vi "niUSRP EX QAM Tx student.vi"() -> ()   [LabVIEW 2020]
doc: "This example <B>requires the Modulation Toolkit</B>.\n\nApplies QAM (Quadrature Amplitude Modulation) to a PN sequence for USRP-based transmission. Continuously transmits a repeating message with a length determined by the PN Sequence Order parameter. \n\nThis example is paired with the example \"niUSRP Ex QAM Rx.vi\", which allows you to establish a Tx / Rx link between two separate USRPs. \n\nTo establish a Tx / Rx link between two USRPs:\n1) Ensure that the Tx and Rx example VIs have matching parameters for Modulation Scheme (M-Ary), Carrier Frequency, and Symbol Rate. Specify the Symbol Rate by setting the combination of the IQ Sampling Rate and the Number of Samples per Symbol parameters.\n2) Choose an IQ Sample Rate that enables sufficient Rx bandwidth.\n3) Set the Tx and / or Rx gain to ensure a sufficient signal to noise ratio on the Receive side. Note: applying too much gain can result in clipping.\n4) Choose a sufficient acquisition frame length that enables the demodulator to lock to the transmitted signal. National Instruments recommends that the acquired frame contain a number of symbols that is at least 20 * M-Ary of the modulation scheme. \n5) Ensure that the Reset Demodulator control is set to True until a solid lock is established. \n6) Install antennas and attenuators that efficiently operate at the carrier frequency you choose."
uses:
  <instrlib>/niUSRP/niUSRP Write Tx Data (CDB Cluster).vi
  <vilib>/addons/Modulation/niDMT.lvlib
panel:
  out "error out":errorcluster
  in  "Enabled Channel":string(combo)="0"
  out "Gain [dB] (actual)":dbl format="%#.6p"
  out "Carrier Frequency \n[Hz] (actual)":dbl=915000000.0 format="%#.6p"
  out "IQ Sampling\nRate [S/sec] (actual)":dbl=500000.0 format="%#.6p"
  in  "Active Antenna":string(combo)="TX1"
  in  "Gain [dB]":dbl format="%#.6p"
  in  "Carrier\nFrequency [Hz]":dbl=915000000.0 format="%#.6p"
  in  "IQ Sampling\nRate [S/sec]":dbl=500000.0 format="%#.6p"
  in  "Device Name":refnum<k15>="192.168.10.5"
  out "Frame Length [samples]":i32=2044
  in  "Pn Sequence Order":i32=13
  in  "Filter Parameters":T1={"Alpha"=0.5, "Filter Length"=6, "TX Filter"=enum."Root Raised Cos"} caption="Pulse Shaping Filter" {"Alpha" format="%.2f"}
  in  "QAM M-Ary":enum16{"4", "8", "16", "32", "64", "128", "256"}(ring)=enum."16"
  out "Symbol Rate [symbols/sec]":dbl=500000.0 format="%#.6p"
  in  "Samples Per Symbol":i32=4 min=2 step=2
  in  "Stop":bool
  out "Constellation Graph":T2(graph) caption="Tx Signal Constellation"
  # "Note:\nFrame size (samples per write) =\n (2^Pn Sequence Order) * Samples Per Symbol.\nUse Pn Sequence Order of 12 when using a 1 Gb Ethernet connection on a USRP RIO device. This prevents underflows by implicitly choosing \na frame size close to the ideal frame size for Ethernet connection. Refer to the \"Data Streaming Performance Tips\" section in the NI-USRP Help at ni.com/manuals for more information."
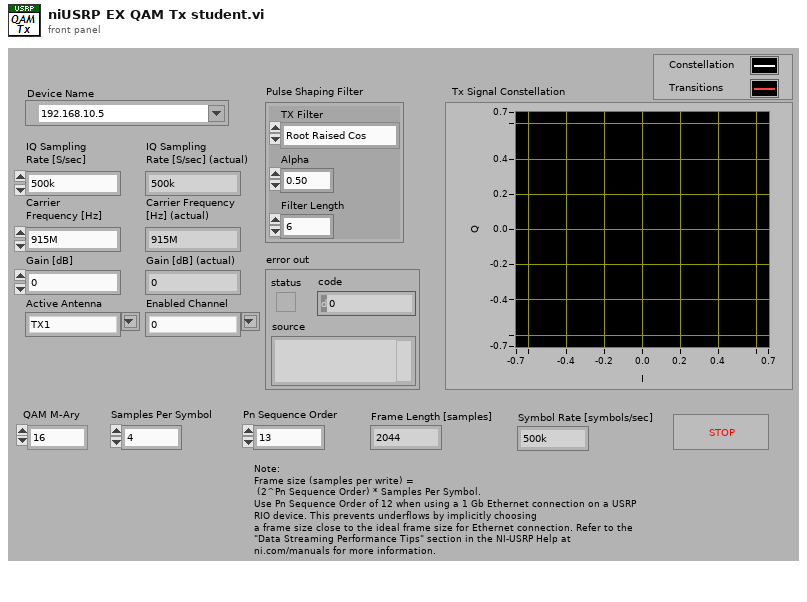
[diagram p1: front panel]
types:
  T1 = cluster{"Alpha":dbl, "Filter Length":i32, "TX Filter":enum16{"none", "Raised Cosine", "Root Raised Cos", "Gaussian"}}
  T2 = cluster{"constellation":dbl[], "oversampled data":dbl[]}[]
  T3 = enum32{"PN sequence", "User-defined pattern", "Read from file"}
  T4 = typedef "niAMT.lvlib/Complex Data Waveform.ctl" = cluster{"t0":dbl, "dt":dbl, "Y":cdb[]}
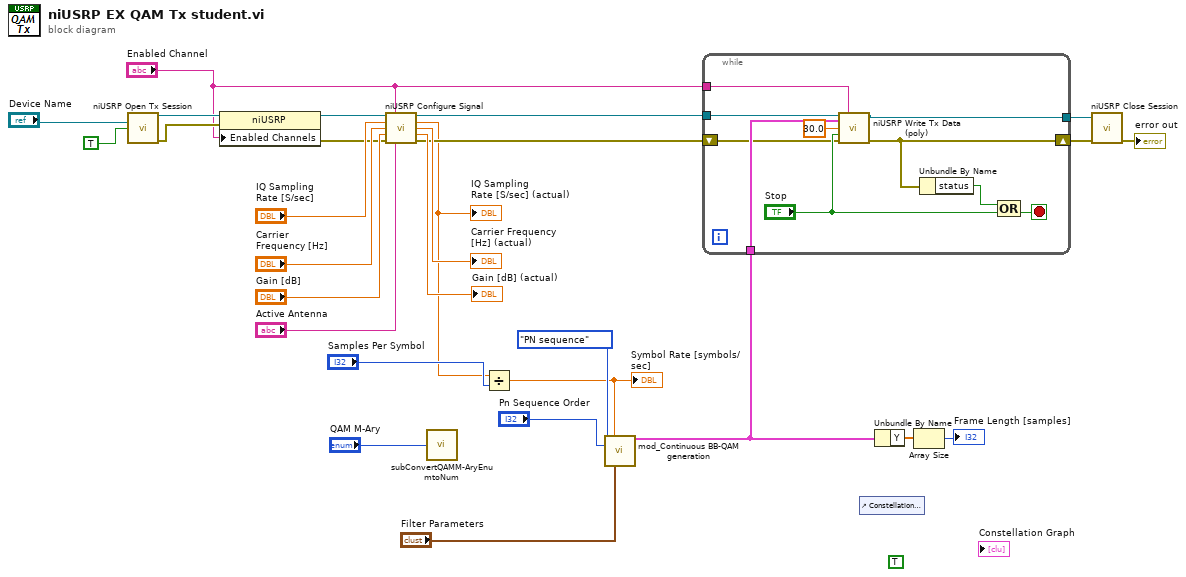
[diagram p0: block diagram]
diagram:
  (unwired) TRUE ("autoscale")
  n1 = call <instrlib>:"niUSRP Open Tx Session.vi"("device names"="Device Name", "reset"=TRUE) -> ("session handle out"=w6:refnum<k15>, "error out"=w4:errorcluster)  [unwired: 12 in]
  n2 = property class="niUSRP"(reference=w6, error in=w4, "Enabled Channels"="Enabled Channel") -> (reference out=w5:refnum<k15>, error out=w3:errorcluster)
  n3 = call <instrlib>:"niUSRP Configure Signal.vi"("session handle"=w5, "channel list"="Enabled Channel", "IQ rate"="IQ Sampling\nRate [S/sec]", "carrier frequency"="Carrier\nFrequency [Hz]", "gain"="Gain [dB]", "error in (no error)"=w3, "active antenna"="Active Antenna") -> ("session handle out"=w9:refnum<k15>, "coerced IQ rate"=w7:dbl, "coerced carrier frequency"=→"Carrier Frequency \n[Hz] (actual)":dbl, "coerced gain"=→"Gain [dB] (actual)":dbl, "error out"=w8:errorcluster)  [unwired: 4 in]
  "IQ Sampling\nRate [S/sec] (actual)" <- w7
  n4 = call "subConvertQAMM-AryEnumtoNum.vi"("QAM M-ary"="QAM M-Ary") -> ()  [unwired: 1 out]
  n5 = Divide(x=w7, y="Samples Per Symbol") -> (x/y=w25:dbl)
  "Symbol Rate [symbols/sec]" <- w25
  n6 = call <vilib>:"mod_Continuous BB-QAM generation.vi"("Bit stream"=T3."PN sequence", "Symbol Rate, Hz"=w25, "PN Sequence Order"="Pn Sequence Order", "filter parameters"="Filter Parameters") -> ("output complex waveform"=w23:T4)  [unwired: 7 in, 4 out]
  n7 = while {
    tunnel: [w36] -> w20
    tunnel: w9 -> [w38]
    shift-right: [w29] -> w19
    shift-left: w8 -> [w32]
    tunnel: w23 -> [w37]
    tunnel: "Enabled Channel" -> [w31]
    stop <- w33 stop-if-true
    n8 = call-poly <instrlib>:"niUSRP Write Tx Data (poly).vi"("session handle"=w38, "channel list"=w31, "data"=w37, "timeout"=30.0, "end of data?"="Stop", "error in (no error)"=w32) -> ("session handle out"=w36:refnum<k15>, "error out"=w29:errorcluster)  [unwired: 8 in]
    n9 = Unbundle By Name(w29) -> ("status"=w35:bool)
    n10 = Compound Arithmetic op=OR(w35, "Stop") -> (w33:bool)
  }
  n11 = control-ref of="Constellation Graph"() -> ()  [unwired: 1 out]
  n12 = Unbundle By Name(w23) -> ("Y"=w28:cdb[])
  n13 = Array Size(array=w28) -> (size(s)=→"Frame Length [samples]":i32)
  n14 = call <instrlib>:"niUSRP Close Session.vi"("session handle"=w20, "error in (no error)"=w19) -> ("error out"=→"error out":errorcluster)  [unwired: 13 in]
